vi "Start.vi"(8 "error in (no error)":errorcluster, 11 "Module Config Selector":i16) -> (0 "error out":errorcluster)   [LabVIEW 2017, in "BOP_VibAPI_4.lvlib"]
uses:
  <vilib>/addons/InsightCM/Devices/Shared/Cms/Fpga/Acquisition/source/subVIs/VibAPI_4/BOP_VibAPI_4.lvlib
  <vilib>/rvi/eio/common/nirviEmuTemplateMethod_errors.vi
  <vilib>/eio/EIONode/EIONode.xnode
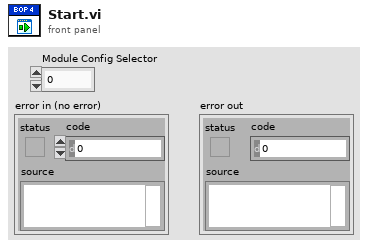
[diagram p1: front panel]
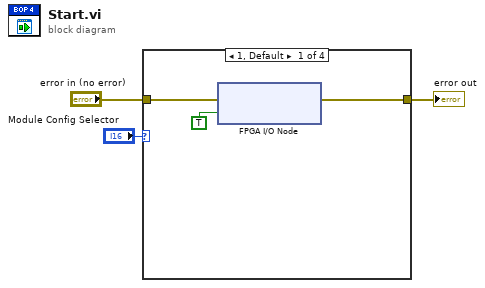
[diagram p0: block diagram]
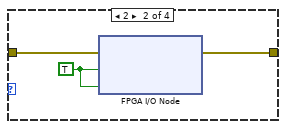
[diagram p2: hidden frame]
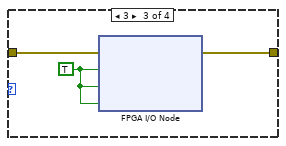
[diagram p3: hidden frame]
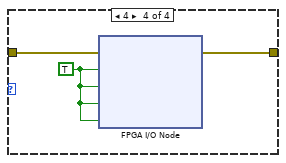
[diagram p4: hidden frame]
diagram:
  n1 = case shown="1, Default" "Module Config Selector" {
    tunnel: "error in (no error)" -> [w5 w8 w11 w14]
    tunnel: [w6 w9 w12 w15] -> w2
    frame 1, Default {
      n2 = xnode "FPGA I/O Node"("error in"=w5, "Mod1/Start"=TRUE) -> ("error out"=w6:errorcluster)  [unwired: 1 in, 1 out]
    }
    frame 2 {
      w7 = TRUE
      n3 = xnode "FPGA I/O Node"("error in"=w8, "Mod1/Start"=w7, "Mod2/Start"=w7) -> ("error out"=w9:errorcluster)  [unwired: 2 in, 2 out]
    }
    frame 3 {
      w10 = TRUE
      n4 = xnode "FPGA I/O Node"("error in"=w11, "Mod1/Start"=w10, "Mod2/Start"=w10, "Mod3/Start"=w10) -> ("error out"=w12:errorcluster)  [unwired: 3 in, 3 out]
    }
    frame 4 {
      w13 = TRUE
      n5 = xnode "FPGA I/O Node"("error in"=w14, "Mod1/Start"=w13, "Mod2/Start"=w13, "Mod3/Start"=w13, "Mod4/Start"=w13) -> ("error out"=w15:errorcluster)  [unwired: 4 in, 4 out]
    }
  }
  "error out" <- w2
